vi "Durability_will_2012_07_02.vi"() -> ()   [LabVIEW 2011]
uses:
  <vilib>/DAQmx/write.llb/DAQmx Write (Counter Time 1Chan 1Samp).vi
  <vilib>/DAQmx/read.llb/DAQmx Read (Analog 1D Wfm NChan NSamp).vi
  <vilib>/express/express shared/ex_Modify Signal Name.vi
  <vilib>/measure/madcrms.llb/Basic Averaged DC-RMS for 1 Chan.vi
  <vilib>/DAQmx/miscellaneous.llb/DAQmx Fill In Error Info.vi
  <vilib>/measure/madcrms.llb/Averaged DC-RMS for N Chan.vi
  <vilib>/express/express arith-compare/Formula/XNode/ExpressFormulaBlockNode.xnode
  <vilib>/measure/NI_MAPro.lvlib
panel:
  out "Waveform Graph":dynamicdata(graph)
  in  "Filename 2":path=path "test.lvm" caption="Filename"
  in  "Filename":path=path "test.lvm"
  out "RPM Graph":dbl(graph)
  out "Motor RPM":dbl format="%#.0f"
  out "Motor Power (watts)":dbl format="%#.4f"
  out "Power to MC1 (watts)":dbl format="%#.4f"
  out "Voltage to MC1 (volts)":dbl format="%#.4f"
  out "Current to MC1  (amps)":dbl format="%#.4f"
  in  "Manual Start":bool
  in  "Power \nSetting":i8(slide) min=0 max=100 step=10 scale=0.0..100.0
  out "Power Setting (%)":dbl format="%#.2f"
  out "Motor Temp (F)":dbl format="%.1f"
  out "Tank Temp (F)":dbl format="%.1f"
  in  "Quit 4":bool
  out "Motor Power Over Time":dbl(graph)
  out "Phase to Phase Voltage":waveform(dbl)(graph)
  out "Phase Current":waveform(dbl)(graph)
  # "Motor Power and RPM"
  # "Temperature"
  # "MC1"
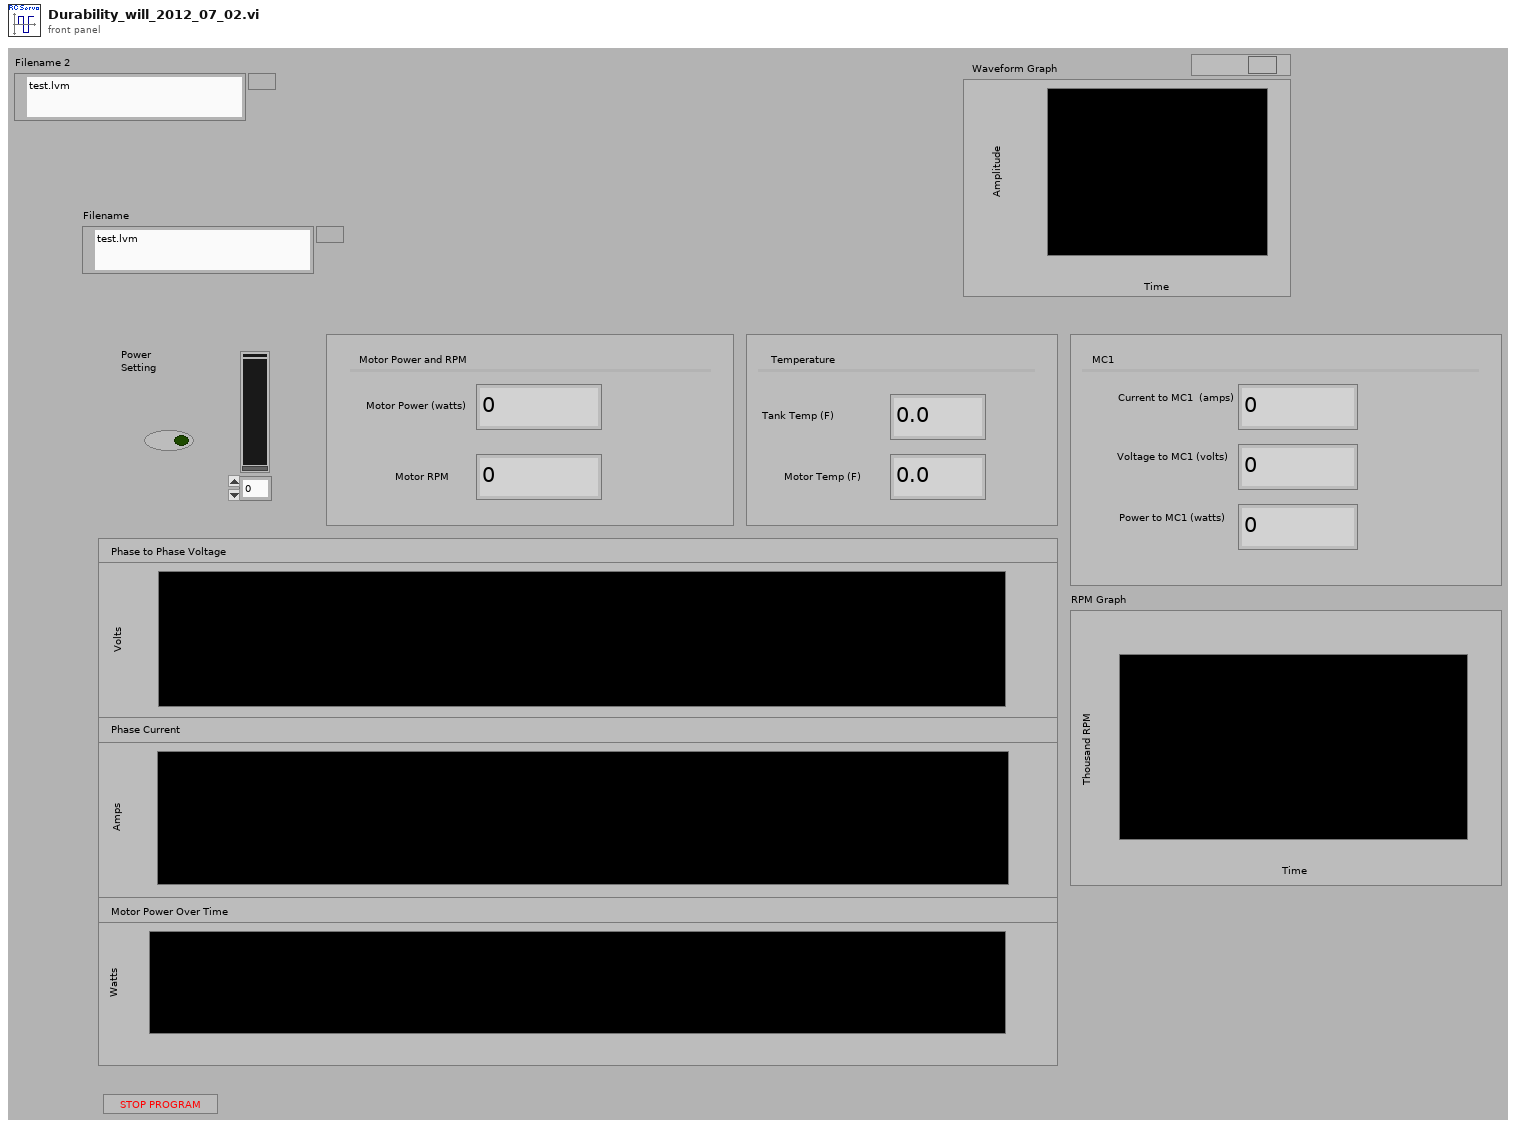
[diagram p1: front panel]
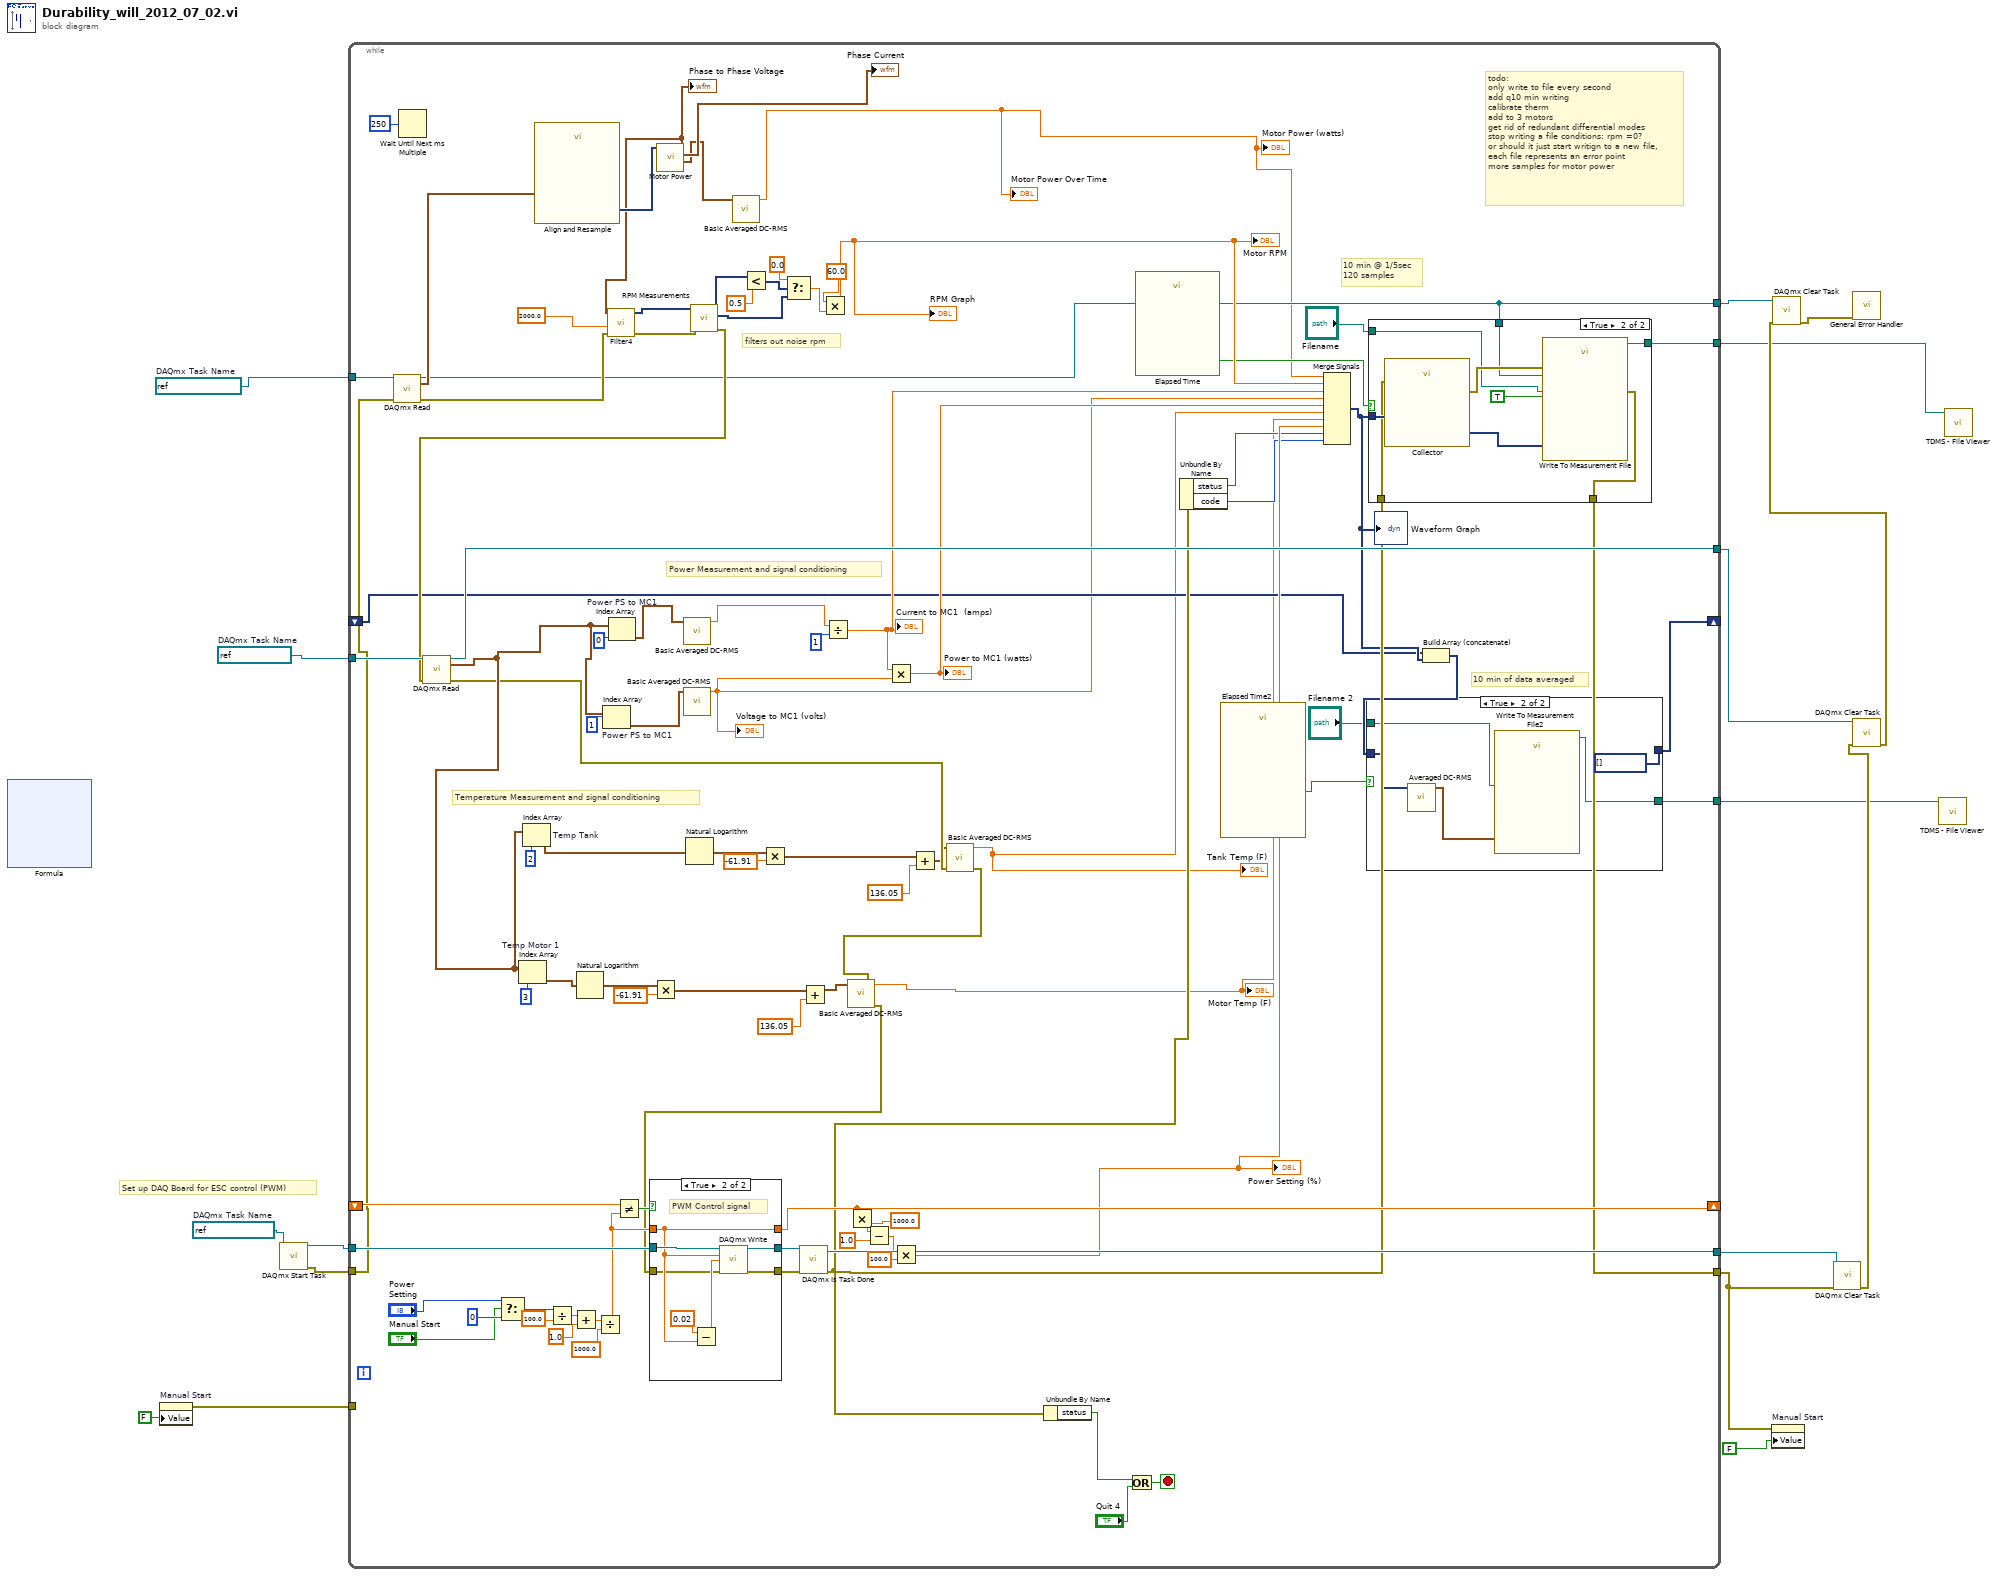
[diagram p0: block diagram]
diagram:
  w8 = refnum<k21> "PWM Signal"  # DAQmx Task Name
  w13 = refnum<k21> "MC Power"  # DAQmx Task Name
  w14 = refnum<k21> "Motor Power"  # DAQmx Task Name
  # "Set up DAQ Board for ESC control (PWM)"
  n1 = xnode "Formula"() -> ()  [unwired: 2 in, 2 out]
  n2 = property on="Manual Start" class="Bool (strict)"("Value"=FALSE ("Run Motor")) -> (error out=w11:errorcluster)  [unwired: 2 in, 1 out]
  n3 = call <vilib>:"DAQmx Start Task.vi"("task/channels in"=w8) -> ("task out"=w7:refnum<k21>, "error out"=w6:errorcluster)  [unwired: 13 in]
  n4 = while {
    tunnel: [w111] -> w17
    tunnel: [w44] -> w9
    tunnel: w7 -> [w109]
    shift-right: [w92] -> _
    shift-left: _ -> [w100]
    tunnel: w13 -> [w87]
    tunnel: [w86] -> w16
    tunnel: [w43] -> w15
    tunnel: w14 -> [w73]
    tunnel: w11 -> [_]
    tunnel: w6 -> [w66]
    shift-right: [w37] -> _
    shift-left: _ -> [w39]
    tunnel: [w36] -> w2
    tunnel: [w33] -> w1
    stop <- w69 stop-if-true
    # "10 min of data averaged"
    # "todo:\nonly write to file every second\nadd q10 min writing\ncalibrate therm\nadd to 3 motors\nget rid of redundant differential modes\nstop writing a file conditions: rpm =0?\nor should it just start writign to a new file,\neach file represents an error point\nmore samples for motor power"
    # "filters out noise rpm"
    # "10 min @ 1/5sec\n120 samples"
    # "Power Measurement and signal conditioning"
    # "Temperature Measurement and signal conditioning"
    n5 = call-poly <vilib>:"DAQmx Read.vi"("task/channels in"=w73, "error in"=w66) -> ("task out"=w43:refnum<k21>, "data"=w48:waveform(dbl)[], "error out"=w83:errorcluster)  [unwired: 11 in]
    n6 = Wait Until Next ms Multiple(millisecond multiple=u32 250) -> ()  [unwired: 1 out]
    n7 = Select(t="Power \nSetting", s="Manual Start", f=i8 0) -> (s? t:f=w98:i8)
    n8 = call "Align and Resample"("Signals"=w48) -> ("Resampled Signals"=w49:dynamicdata)  [unwired: 8 in, 2 out]
    n9 = Divide(x=w98, y=100.0) -> (x/y=w104:dbl)
    n10 = Add(x=w104, y=1.0 ("x/y")) -> (x+y=w102:dbl)
    n11 = Divide(x=w102, y=1000.0) -> (x/y=w101:dbl)
    n12 = Not Equal?(x=w100, y=w101) -> (x != y?=w110:bool)
    n13 = call "Motor Power.vi"("data"=w49) -> ("Waveform"=w32:waveform(dbl), "Phase Current"=→"Phase Current":waveform(dbl), "Phase to Phase Voltage"=w46:waveform(dbl))  [unwired: 7 in, 1 out]
    "Phase to Phase Voltage" <- w46
    n14 = call "Filter4"("error in (no error)"=w83, "Lower Cut-Off"=2000.0 ("LowPass Filter CutOff [Hz]"), "Signal"=w46) -> ("error out"=w84:errorcluster, "Filtered Signal"=w75:dynamicdata)  [unwired: 7 in]
    n15 = call "RPM Measurements"("error in (no error)"=w84, "Signals"=w75) -> ("error out"=w68:errorcluster, "Frequency"=w79:dynamicdata, "Amplitude"=w76:dynamicdata)  [unwired: 7 in]
    n16 = call-poly <vilib>:"DAQmx Read.vi"("task/channels in"=w87, "error in"=w68) -> ("task out"=w86:refnum<k21>, "data"=w25:waveform(dbl)[], "error out"=w23:errorcluster)  [unwired: 11 in]
    n17 = Index Array "Temp Motor 1"(array=w25, index=3) -> (element=w61:waveform(dbl))
    n18 = Index Array "Temp Tank"(array=w25, index=2) -> (element=w26:waveform(dbl))
    n19 = Natural Logarithm(1:w61) -> (0:w65:waveform(dbl))
    n20 = Index Array "Power PS to MC1"(array=w25, index=1) -> (element=w28:waveform(dbl))
    n21 = Index Array "Power PS to MC1"(array=w25, index=0) -> (element=w30:waveform(dbl))
    n22 = Multiply(x=w65, y=-61.91) -> (x*y=w63:waveform(dbl))
    n23 = call-poly <vilib>:"Basic Averaged DC-RMS.vi"("signal in"=w30) -> ("DC value"=w29:dbl)  [unwired: 7 in, 3 out]
    n24 = call-poly <vilib>:"Basic Averaged DC-RMS.vi"("signal in"=w28) -> ("DC value"=w27:dbl)  [unwired: 7 in, 3 out]
    "Voltage to MC1 (volts)" <- w27
    n25 = Natural Logarithm(1:w26) -> (0:w60:waveform(dbl))
    n26 = call-poly <vilib>:"Basic Averaged DC-RMS.vi"("signal in"=w32) -> ("DC value"=w31:dbl)  [unwired: 7 in, 3 out]
    "Motor Power Over Time" <- w31
    "Motor Power (watts)" <- w31
    n27 = Less?(x=w76, y=0.5) -> (x < y?=w78:dynamicdata)
    n28 = Multiply(x=w60, y=-61.91) -> (x*y=w58:waveform(dbl))
    n29 = Select(t=0.0, s=w78, f=w79) -> (s? t:f=w81:dbl)
    n30 = Add(x=w63, y=136.05) -> (x+y=w21:waveform(dbl))
    n31 = Multiply(x=60.0, y=w81) -> (x*y=w55:dbl)
    "Motor RPM" <- w55
    "RPM Graph" <- w55
    n32 = Divide(x=w29, y=1) -> (x/y=w54:dbl)
    "Current to MC1  (amps)" <- w54
    n33 = Multiply(x=w54, y=w27) -> (x*y=w53:dbl)
    "Power to MC1 (watts)" <- w53
    n34 = Add(x=w58, y=136.05) -> (x+y=w22:waveform(dbl))
    n35 = call-poly <vilib>:"Basic Averaged DC-RMS.vi"("error in (no error)"=w23, "signal in"=w22) -> ("error out"=w18:errorcluster, "DC value"=w24:dbl)  [unwired: 6 in, 2 out]
    "Tank Temp (F)" <- w24
    n36 = call-poly <vilib>:"Basic Averaged DC-RMS.vi"("error in (no error)"=w18, "signal in"=w21) -> ("error out"=w19:errorcluster, "DC value"=w20:dbl)  [unwired: 6 in, 2 out]
    "Motor Temp (F)" <- w20
    n37 = case shown="True" w110 {
      tunnel: w101 -> [w131 w134]
      tunnel: w109 -> [w132 w138]
      tunnel: [w132 w136] -> w108
      tunnel: [w130 w135] -> w107
      tunnel: [w131 w134] -> w92
      tunnel: w19 -> [w130 w133]
      frame False {
      }
      frame True {
        # "PWM Control signal"
        n38 = Subtract(x=0.02, y=w134) -> (x-y=w137:dbl)
        n39 = call-poly <vilib>:"DAQmx Write.vi"("task/channels in"=w138, "high time"=w134, "low time"=w137, "error in"=w133) -> ("task out"=w136:refnum<k21>, "error out"=w135:errorcluster)  [unwired: 9 in, 1 out]
      }
    }
    n40 = call <vilib>:"DAQmx Is Task Done.vi"("task/channels in"=w108, "error in"=w107) -> ("task out"=w111:refnum<k21>, "error out"=w45:errorcluster)  [unwired: 11 in, 1 out]
    n41 = Multiply(x=w92, y=1000.0) -> (x*y=w93:dbl)
    n42 = Subtract(x=w93, y=1.0) -> (x-y=w96:dbl)
    n43 = Multiply(x=w96, y=100.0) -> (x*y=w52:dbl)
    "Power Setting (%)" <- w52
    n44 = Unbundle By Name(w45) -> ("status"=w67:bool)
    n45 = Or(x=w67, y="Quit 4") -> (x .or. y?=w69:bool)
    n46 = call "Elapsed Time"() -> ("Time has Elapsed"=w42:bool)  [unwired: 12 in, 7 out]
    n47 = Unbundle By Name(w45) -> ("status"=w51:bool, "code"=w50:i32)
    n48 = call "Elapsed Time2"() -> ("Time has Elapsed"=w41:bool)  [unwired: 12 in, 7 out]
    n49 = Merge Signals(w31, w55, w54, w27, w53, w24, w20, w52, w51, w50) -> (w40:dynamicdata)
    "Waveform Graph" <- w40
    n50 = case shown="True" w42 {
      tunnel: w40 -> [_ w129]
      tunnel: w45 -> [w120 w127]
      tunnel: [w120 w125] -> w44
      tunnel: w43 -> [_ w123]
      tunnel: "Filename" -> [w119 w122]
      tunnel: [w119 w121] -> w33
      frame False {
      }
      frame True {
        n51 = call "Collector"("error in (no error)"=w127, "Signals"=w129) -> ("error out"=w126:errorcluster, "Collected Signals"=w128:dynamicdata)  [unwired: 8 in]
        n52 = call "Write To Measurement File"("Signals"=w128, "Reset"=TRUE, "error in (no error)"=w126, "Filename"=w122, "DAQmx Task"=w123) -> ("Filename Out"=w121:path, "error out"=w125:errorcluster)  [unwired: 12 in, 1 out]
      }
    }
    n53 = Build Array (concatenate)(w39, w40) -> (w38:dynamicdata[])
    n54 = case shown="True" w41 {
      tunnel: w38 -> [w113 w117]
      tunnel: [w113 dynamicdata[] []] -> w37
      tunnel: [w112 w115] -> w36
      tunnel: "Filename 2" -> [w112 w114]
      frame False {
      }
      frame True {
        n55 = call-poly <vilib>:"Averaged DC-RMS.vi"("signals in"=w117) -> ("DC value waveforms"=w116:waveform(dbl)[])  [unwired: 6 in, 4 out]
        n56 = call "Write To Measurement File2"("Signals"=w116, "Filename"=w114) -> ("Filename Out"=w115:path)  [unwired: 15 in, 2 out]
      }
    }
  }
  n57 = property on="Manual Start" class="Bool (strict)"(error in=w9, "Value"=FALSE ("Run Motor")) -> ()  [unwired: 1 in, 2 out]
  n58 = call <vilib>:"DAQmx Clear Task.vi"("task in"=w17, "error in"=w9) -> ("error out"=w3:errorcluster)  [unwired: 13 in]
  n59 = call <vilib>:"DAQmx Clear Task.vi"("task in"=w16, "error in"=w3) -> ("error out"=w5:errorcluster)  [unwired: 13 in]
  n60 = call <vilib>:"DAQmx Clear Task.vi"("task in"=w15, "error in"=w5) -> ("error out"=w4:errorcluster)  [unwired: 13 in]
  n61 = call <vilib>:"General Error Handler.vi"("error in (no error)"=w4) -> ()  [unwired: 10 in, 5 out]
  n62 = call <vilib>:"TDMS - File Viewer.vi"("file path"=w2) -> ()  [unwired: 1 in, 6 out]
  n63 = call <vilib>:"TDMS - File Viewer.vi"("file path"=w1) -> ()  [unwired: 1 in, 6 out]
